vi "MCS_OpenSystem.vi"(2 "error in (no error)":errorcluster, 3 "MCS System Locator":string) -> (0 "error out":errorcluster, 1 "System Index Out":u32)   [LabVIEW 2010]
uses:
  <vilib>/SmarAct/MCS/Types/mcsSensorTypes.ctl
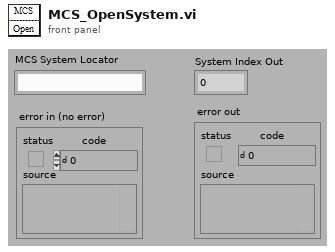
[diagram p1: front panel]
types:
  T1 = typedef "mcsSensorTypes.ctl" = enum32{"SA_NO_SENSOR_TYPE", "SA_S_SENSOR_TYPE", "SA_SR_SENSOR_TYPE", "SA_ML_SENSOR_TYPE", "SA_MR_SENSOR_TYPE", "SA_SP_SENSOR_TYPE", "SA_SC_SENSOR_TYPE", "SA_M25_SENSOR_TYPE", "SA_SR20_SENSOR_TYPE", "SA_M_SENSOR_TYPE", "SA_GC_SENSOR_TYPE", "SA_GD_SENSOR_TYPE", "SA_GE_SENSOR_TYPE", "SA_RA_SENSOR_TYPE", "SA_GF_SENSOR_TYPE", "SA_RB_SENSOR_TYPE", "SA_G605S_SENSOR_TYPE", "SA_G775S_SENSOR_TYPE", "SA_SC500_SENSOR_TYPE", "SA_G955S_SENSOR_TYPE", "SA_SR77_SENSOR_TYPE", "SA_SD_SENSOR_TYPE", "SA_R20ME_SENSOR_TYPE", "SA_SR2_SENSOR_TYPE", "SA_SCD_SENSOR_TYPE", "SA_SRC_SENSOR_TYPE", "SA_SR36M_SENSOR_TYPE", "SA_SR36ME_SENSOR_TYPE", "SA_SR50M_SENSOR_TYPE", "SA_SR50ME_SENSOR_TYPE", "SA_G1045S_SENSOR_TYPE", "SA_G1395S_SENSOR_TYPE", "SA_MD_SENSOR_TYPE", "SA_G935M_SENSOR_TYPE", "SA_SHL20_SENSOR_TYPE", "SA_SCT_SENSOR_TYPE", "SA_SR77T_SENSOR_TYPE", "SA_SR120_SENSOR_TYPE", "SA_LC_SENSOR_TYPE", "SA_LR_SENSOR_TYPE", "SA_LCD_SENSOR_TYPE", "SA_L_SENSOR_TYPE", "SA_LD_SENSOR_TYPE"}
  T2 = enum32{"SA_SENSOR_DISABLED", "SA_SENSOR_ENABLED", "SA_SENSOR_POWERSAVE"}
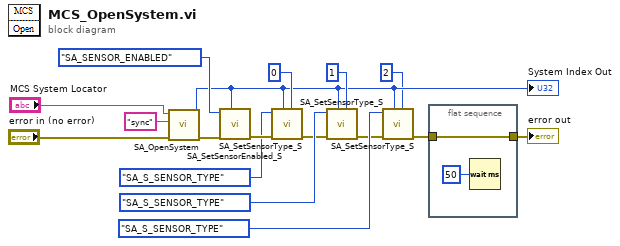
[diagram p0: block diagram]
diagram:
  n1 = call <vilib>:"SA_OpenSystem.vi"("error in (no error)"="error in (no error)", "options"="sync", "systemLocator"="MCS System Locator") -> ("error out"=w13:errorcluster, "systemIndexOut"=w4:u32)  [unwired: 7 in]
  "System Index Out" <- w4
  n2 = call <vilib>:"SA_SetSensorEnabled_S.vi"("systemIndex"=w4, "error in (no error)"=w13, "enabled"=T2."SA_SENSOR_ENABLED") -> ("error out"=w12:errorcluster)  [unwired: 8 in]
  n3 = call <vilib>:"SA_SetSensorType_S.vi"("channelIndex"=u32 0, "systemIndex"=w4, "error in (no error)"=w12, "type"=mcsSensorTypes."SA_S_SENSOR_TYPE") -> ("error out"=w8:errorcluster)  [unwired: 7 in]
  n4 = call <vilib>:"SA_SetSensorType_S.vi"("channelIndex"=u32 1, "systemIndex"=w4, "error in (no error)"=w8, "type"=mcsSensorTypes."SA_S_SENSOR_TYPE") -> ("error out"=w5:errorcluster)  [unwired: 7 in]
  n5 = call <vilib>:"SA_SetSensorType_S.vi"("channelIndex"=u32 2, "systemIndex"=w4, "error in (no error)"=w5, "type"=mcsSensorTypes."SA_S_SENSOR_TYPE") -> ("error out"=w2:errorcluster)  [unwired: 7 in]
  n6 = flat-sequence {
    tunnel: w2 -> [w18]
    tunnel: [w18] -> w1
    frame #0 {
      n7 = Wait (ms)(milliseconds to wait=u32 50) -> ()  [unwired: 1 out]
    }
  }
  "error out" <- w1
